vi "ConfigureSafetyParameter.vi"(0 "axis in":cluster{"keyHandle":u32, "nodeId":u16}={"keyHandle"=0, "nodeId"=1}, 5 "maxFollowingError":u32, 7 "maxProfileVelocity":u32, 9 "maxAcceleration":u32, 11 "error in (no error)":errorcluster) -> (4 "axis out":cluster{"keyHandle":u32, "nodeId":u16}={"keyHandle"=0, "nodeId"=1}, 15 "error out":errorcluster)   [LabVIEW 2019, in "maxonEPOS.lvlib"]
doc: "<B>ConfigureSafetyParameter</B> writes the safety parameters to the device. The parameters for <B>Max Following Error</B>, <B>Max Profile Velocity</B> and <B>Max Acceleration</B> will be adjusted."
uses:
  Examples/maxonEPOS.lvlib
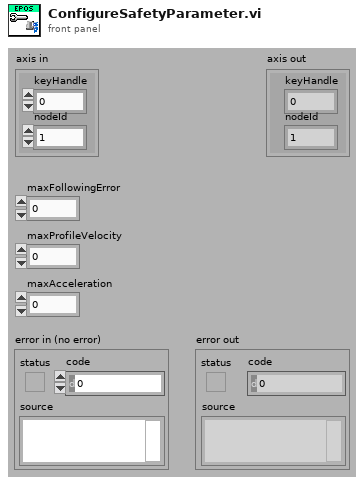
[diagram p1: front panel]
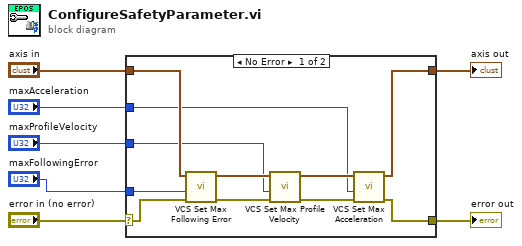
[diagram p0: block diagram]
diagram:
  n1 = case shown="No Error" "error in (no error)" {
    selector: "error in (no error)" -> [w18 w20]
    tunnel: [w15 w20] -> w6
    tunnel: [w14 w19] -> w5
    tunnel: "axis in" -> [w11 w19]
    tunnel: "maxFollowingError" -> [w10 _]
    tunnel: "maxProfileVelocity" -> [w9 _]
    tunnel: "maxAcceleration" -> [w8 _]
    frame No Error {
      n2 = call "VCS Set Max Following Error.vi"("error in (no error)"=w18, "maxFollowingError"=w10, "axis in"=w11) -> ("error out"=w17:errorcluster, "axis out"=w12:cluster{"keyHandle":u32, "nodeId":u16})  [unwired: 7 in]
      n3 = call "VCS Set Max Profile Velocity.vi"("error in (no error)"=w17, "maxProfileVelocity"=w9, "axis in"=w12) -> ("error out"=w16:errorcluster, "axis out"=w13:cluster{"keyHandle":u32, "nodeId":u16})  [unwired: 7 in]
      n4 = call "VCS Set Max Acceleration.vi"("error in (no error)"=w16, "maxAcceleration"=w8, "axis in"=w13) -> ("error out"=w15:errorcluster, "axis out"=w14:cluster{"keyHandle":u32, "nodeId":u16})  [unwired: 7 in]
    }
    frame Error {
    }
  }
  "error out" <- w6
  "axis out" <- w5
